vi "Detect BOM.vi"(11 "String":string) -> (1 "BOM Found":bool, 2 "Encoding":T1)   [LabVIEW 2020, in "G-Unicode.lvlib"]
doc: "Checks <b>String</b> for a Byte Order Mark (BOM). If a BOM is present, <b>BOM Found</b> will be TRUE, and <b>Encoding</b> will be set to the corresponding encoding indicated by the BOM. If no BOM is found, BOM Found will be FALSE and Encoding will be Unknown."
uses:
  G-Unicode.lvlib
  Controls/String Encoding.ctl
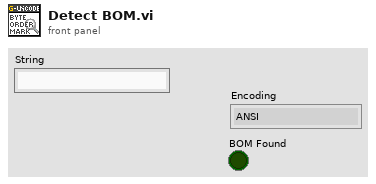
[diagram p1: front panel]
types:
  T1 = typedef "G-Unicode.lvlib/String Encoding.ctl" = enum16{"ANSI", "UTF-8", "UTF-16LE", "UTF-16BE", "Unknown"}
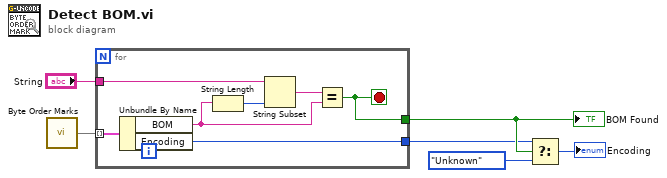
[diagram p0: block diagram]
diagram:
  n1 = call "Byte Order Marks.vi"() -> ("BOMs"=w1:map{T1, string})
  n2 = for {
    tunnel: "String" -> [w11]
    tunnel: [w7] -> w5
    tunnel: [w12] -> w4
    tunnel: w1 -> [w13] mode=indexing
    stop <- w7 stop-if-true
    n3 = Unbundle By Name(w13) -> ("BOM"=w8:string, "Encoding"=w12:T1)
    n4 = String Length(string=w8) -> (length=w10:i32)
    n5 = String Subset(string=w11, length (rest)=w10) -> (substring=w9:string)  [unwired: 1 in]
    n6 = Equal?(x=w9, y=w8) -> (x = y?=w7:bool)
  }
  "BOM Found" <- w5
  n7 = Select(t=w4, s=w5, f=String_Encoding."Unknown") -> (s? t:f=→"Encoding":T1)
